vi "Update Water Level.vi"(8 "error in (no error)":cluster{"状态":bool, "代码":i32, "源":string} caption="错误输入（无错误）", 10 "水位":dbl, 11 "蒸发冷却器":refnum<class "Evaporative Cooler.lvclass">) -> (0 "error out":cluster{"状态":bool, "代码":i32, "源":string} caption="错误输出", 3 "蒸发冷却器":refnum<class "Evaporative Cooler.lvclass">)   [LabVIEW 2013, in "Evaporative Cooler.lvlib" / "Evaporative Cooler.lvclass"]
doc: "该方法向控制器发送消息，通知水槽的水位信息。"
uses:
  Evaporative Cooler/Evaporative Cooler/Evaporative Cooler.lvclass
  <vilib>/ActorFramework/Message Enqueuer/Message Enqueuer.lvclass
  Cooler.lvclass/Cooler.ctl
  Evaporative Cooler Controller/Update Water Level Msg/Update Water Level Msg.lvclass/Update Water Level Msg.ctl
  <vilib>/ActorFramework/Message Enqueuer/Message Enqueuer.lvclass/Message Enqueuer.ctl
  <vilib>/ActorFramework/Message Enqueuer/Enqueue.vi
  <vilib>/ActorFramework/Message Priority Queue/Priority Enqueue.vi
  Evaporative Cooler Controller/Update Water Level Msg/Update Water Level Msg.lvclass
  Cooler.lvclass
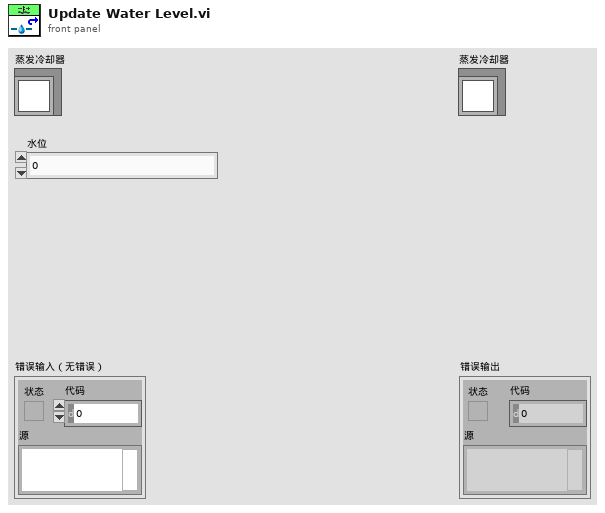
[diagram p1: front panel]
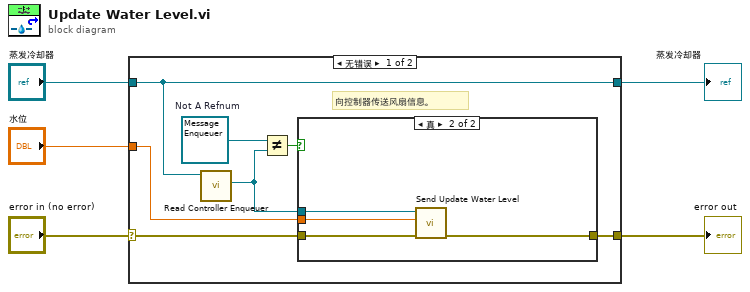
[diagram p0: block diagram]
diagram:
  n1 = case shown="无错误" "error in (no error)" {
    selector: "error in (no error)" -> [w11 w19]
    tunnel: [w10 w19] -> w4
    tunnel: [w12 w18] -> w2
    tunnel: "蒸发冷却器" -> [w12 w18]
    tunnel: "水位" -> [w6 _]
    frame No Error {
      w8 = refnum<class "Message Enqueuer.lvclass"> refnum  # Not A Refnum
      # "向控制器传送风扇信息。"
      n2 = call "Read Controller Enqueuer.vi"("冷却器"=w12) -> ("控制器待入队列"=w9:refnum<class "Message Enqueuer.lvclass">)  [unwired: 10 in]
      n3 = Not Equal?(x=w8, y=w9) -> (x != y?=w7:bool)
      n4 = case shown="真" w7 {
        tunnel: w9 -> [_ w17]
        tunnel: w11 -> [w13 w16]
        tunnel: [w13 w15] -> w10
        tunnel: w6 -> [_ w14]
        frame False {
        }
        frame True {
          n5 = call "Send Update Water Level.vi"("error in (no error)"=w16, "水位"=w14, "消息待入队列"=w17) -> ("error out"=w15:cluster{"状态":bool, "代码":i32, "源":string})  [unwired: 8 in]
        }
      }
    }
    frame Error {
    }
  }
  "error out" <- w4
  "蒸发冷却器" <- w2
